vi "get_lines_per_frame.vi"(8 "error in (no error)":errorcluster, 11 "ScanModeCN090721ThreeDScan in":refnum<class "ImagingModeDL100901FlexTrajectory.lvclass">) -> (0 "error out":errorcluster, 2 "lines per frame":i32, 3 "ScanModeCN090721ThreeDScan out":refnum<class "ImagingModeDL100901FlexTrajectory.lvclass">)   [LabVIEW 2010, in "ImagingModeDL100901FlexTrajectory.lvclass"]
uses:
  ImagingModeDL100901FlexTrajectory.lvclass
  ImagingModeDL100901FlexTrajectory.lvclass/ImagingModeDL100901FlexTrajectory.ctl
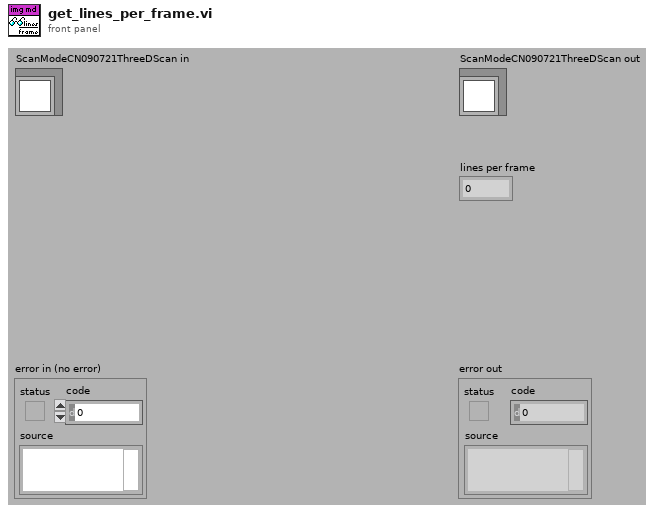
[diagram p1: front panel]
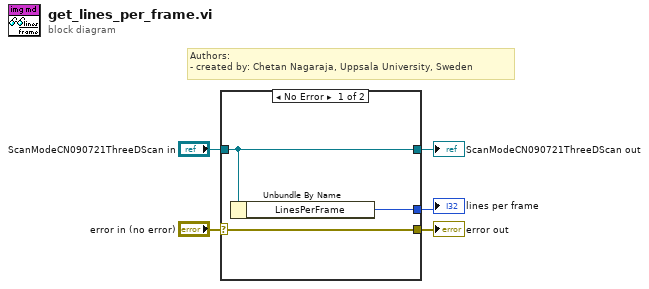
[diagram p0: block diagram]
diagram:
  # "Authors: \n- created by: Chetan Nagaraja, Uppsala University, Sweden"
  n1 = case shown="No Error" "error in (no error)" {
    selector: "error in (no error)" -> [w8 w10]
    tunnel: [w8 w10] -> w4
    tunnel: [w7 w9] -> w2
    tunnel: "ScanModeCN090721ThreeDScan in" -> [w7 w9]
    tunnel: [w6 _] -> w1
    frame No Error {
      n2 = Unbundle By Name(w7) -> ("LinesPerFrame"=w6:i32)
    }
    frame Error {
    }
  }
  "error out" <- w4
  "ScanModeCN090721ThreeDScan out" <- w2
  "lines per frame" <- w1
